vi "NI OCR-Detect Characters Setting.vi"(8 "error in":errorcluster, 11 "Buffer Data In":T3={"VI Refnum"=refnum, "Src Image"="NI OCR-Src Image", "Dst Image"="NI OCR-Dst Image", "Ctl Refnum []"=[refnum, refnum, refnum], "Ctl Label"=["Detect Characters", "Display Image", "Import Picture"], "User Event"=refnum, "Event Registration Refnum"=refnum, "Timeout"=-1, "IMAQ OCR Session"=refnum, "Objects"=[], "ROI Descriptor"={"Global Rectangle"=[], "Contours"=[]}, "Settings"={"Objects"=0, "Threshold"=128, "Reject Border"=FALSE, "Fill Holes"=FALSE, "Min Object Size"=FALSE, "Min Size"=3, "Max Object Size"=FALSE, "Max Size"=100, "Show Search Area"=FALSE, "Show Center"=TRUE, "Show Bounding Box"=TRUE}} {"Settings"."Objects" items=["Bright Objects", "Dark Objects"]; "Settings"."Threshold" min=1 max=999999999 step=1; "Settings"."Max Size" min=1 max=999999999 step=1; "Settings"."Min Size" min=1 max=999999999 step=1; "ROI Descriptor"."Contours"."Type" items=["No Selection", "Point", "Line", "Rectangle", "Oval", "Polygon", "Freehand Region", "Annulus", "Unused2", "Unused3", "Broken Line", "Freehand Line", "Rotated Rectangle"]; "Objects"."Aspect Ratio" format="%.2f"; "Objects"."Orientation" format="%.2f"; "Objects"."Area" format="%.2f"; "Objects"."Object Center"."Y" format="%.2f"; "Objects"."Object Center"."X" format="%.2f"}) -> (0 "error out":errorcluster, 2 "OK?":bool, 3 "Buffer Data Out":T3={"VI Refnum"=refnum, "Src Image"="NI OCR-Src Image", "Dst Image"="NI OCR-Dst Image", "Ctl Refnum []"=[refnum, refnum, refnum], "Ctl Label"=["Detect Characters", "Display Image", "Import Picture"], "User Event"=refnum, "Event Registration Refnum"=refnum, "Timeout"=-1, "IMAQ OCR Session"=refnum, "Objects"=[{"Object Center"={"X"=111.53468, "Y"=84.57803}, "Bounding Box"={"X Left"=95, "Y Top"=62, "X Right"=124, "Y Bottom"=108}, "Area"=692.0, "Orientation"=88.71199, "Aspect Ratio"=0.6304348, "Nb Holes"=0}, {"Object Center"={"X"=74.43038, "Y"=89.12658}, "Bounding Box"={"X Left"=60, "Y Top"=64, "X Right"=89, "Y Bottom"=110}, "Area"=632.0, "Orientation"=97.4022, "Aspect Ratio"=0.6304348, "Nb Holes"=0}, {"Object Center"={"X"=147.98517, "Y"=88.570015}, "Bounding Box"={"X Left"=132, "Y Top"=66, "X Right"=160, "Y Bottom"=112}, "Area"=607.0, "Orientation"=87.522575, "Aspect Ratio"=0.6086956, "Nb Holes"=0}, {"Object Center"={"X"=179.27258, "Y"=95.40412}, "Bounding Box"={"X Left"=168, "Y Top"=68, "X Right"=197, "Y Bottom"=114}, "Area"=631.0, "Orientation"=112.89326, "Aspect Ratio"=0.6304348, "Nb Holes"=1}, {"Object Center"={"X"=271.875, "Y"=72.375}, "Bounding Box"={"X Left"=270, "Y Top"=69, "X Right"=274, "Y Bottom"=78}, "Area"=24.0, "Orientation"=99.49205, "Aspect Ratio"=0.44444445, "Nb Holes"=0}, {"Object Center"={"X"=217.32158, "Y"=92.65162}, "Bounding Box"={"X Left"=203, "Y Top"=70, "X Right"=232, "Y Bottom"=116}, "Area"=709.0, "Orientation"=79.66425, "Aspect Ratio"=0.6304348, "Nb Holes"=0}, {"Object Center"={"X"=248.96008, "Y"=100.51471}, "Bounding Box"={"X Left"=241, "Y Top"=73, "X Right"=269, "Y Bottom"=118}, "Area"=476.0, "Orientation"=108.11947, "Aspect Ratio"=0.62222224, "Nb Holes"=0}], "ROI Descriptor"={"Global Rectangle"=[], "Contours"=[]}, "Settings"={"Objects"=0, "Threshold"=128, "Reject Border"=FALSE, "Fill Holes"=FALSE, "Min Object Size"=FALSE, "Min Size"=3, "Max Object Size"=FALSE, "Max Size"=100, "Show Search Area"=FALSE, "Show Center"=TRUE, "Show Bounding Box"=TRUE}} {"Settings"."Objects" items=["Bright Objects", "Dark Objects"]; "Settings"."Threshold" min=1 max=999999999 step=1; "Settings"."Max Size" min=1 max=999999999 step=1; "Settings"."Min Size" min=1 max=999999999 step=1; "ROI Descriptor"."Contours"."Type" items=["No Selection", "Point", "Line", "Rectangle", "Oval", "Polygon", "Freehand Region", "Annulus", "Unused2", "Unused3", "Broken Line", "Freehand Line", "Rotated Rectangle"]; "Objects"."Aspect Ratio" format="%.2f"; "Objects"."Orientation" format="%.2f"; "Objects"."Area" format="%.2f"; "Objects"."Object Center"."Y" format="%.2f"; "Objects"."Object Center"."X" format="%.2f"})   [LabVIEW 2016]
uses:
  Data Def/NI OCR-Buffer Data.ctl
  <vilib>/vision/Image Controls.llb/IMAQ Image.ctl
  Data Def/NI OCR-User Event Data.ctl
  <vilib>/vision/OCR.llb/IMAQ OCR Session.ctl
  <vilib>/Utility/miscctls.llb/LVPointTypeDef.ctl
  Data Def/NI OCR-Detect Characters State.ctl
panel:
  in  "Cancel":bool
  in  "OK":bool
  in  "Setting":T1={"Objects"=1, "Threshold"=128.0, "Ignore Objects touching Image Borders"=FALSE, "Fill Holes within Objects"=FALSE, "Minimum Object Size"=FALSE, "Min Size(Pixels)"=0.0, "Maximum Object Size"=FALSE, "Max Size(Pixels)"=1000.0, "Show Search Area"=TRUE, "Show Center"=TRUE, "Show Bounding Box"=TRUE} {"Objects" items=["Bright Objects", "Dark Objects"]}
  out "Display Image":T2(plugin-control)
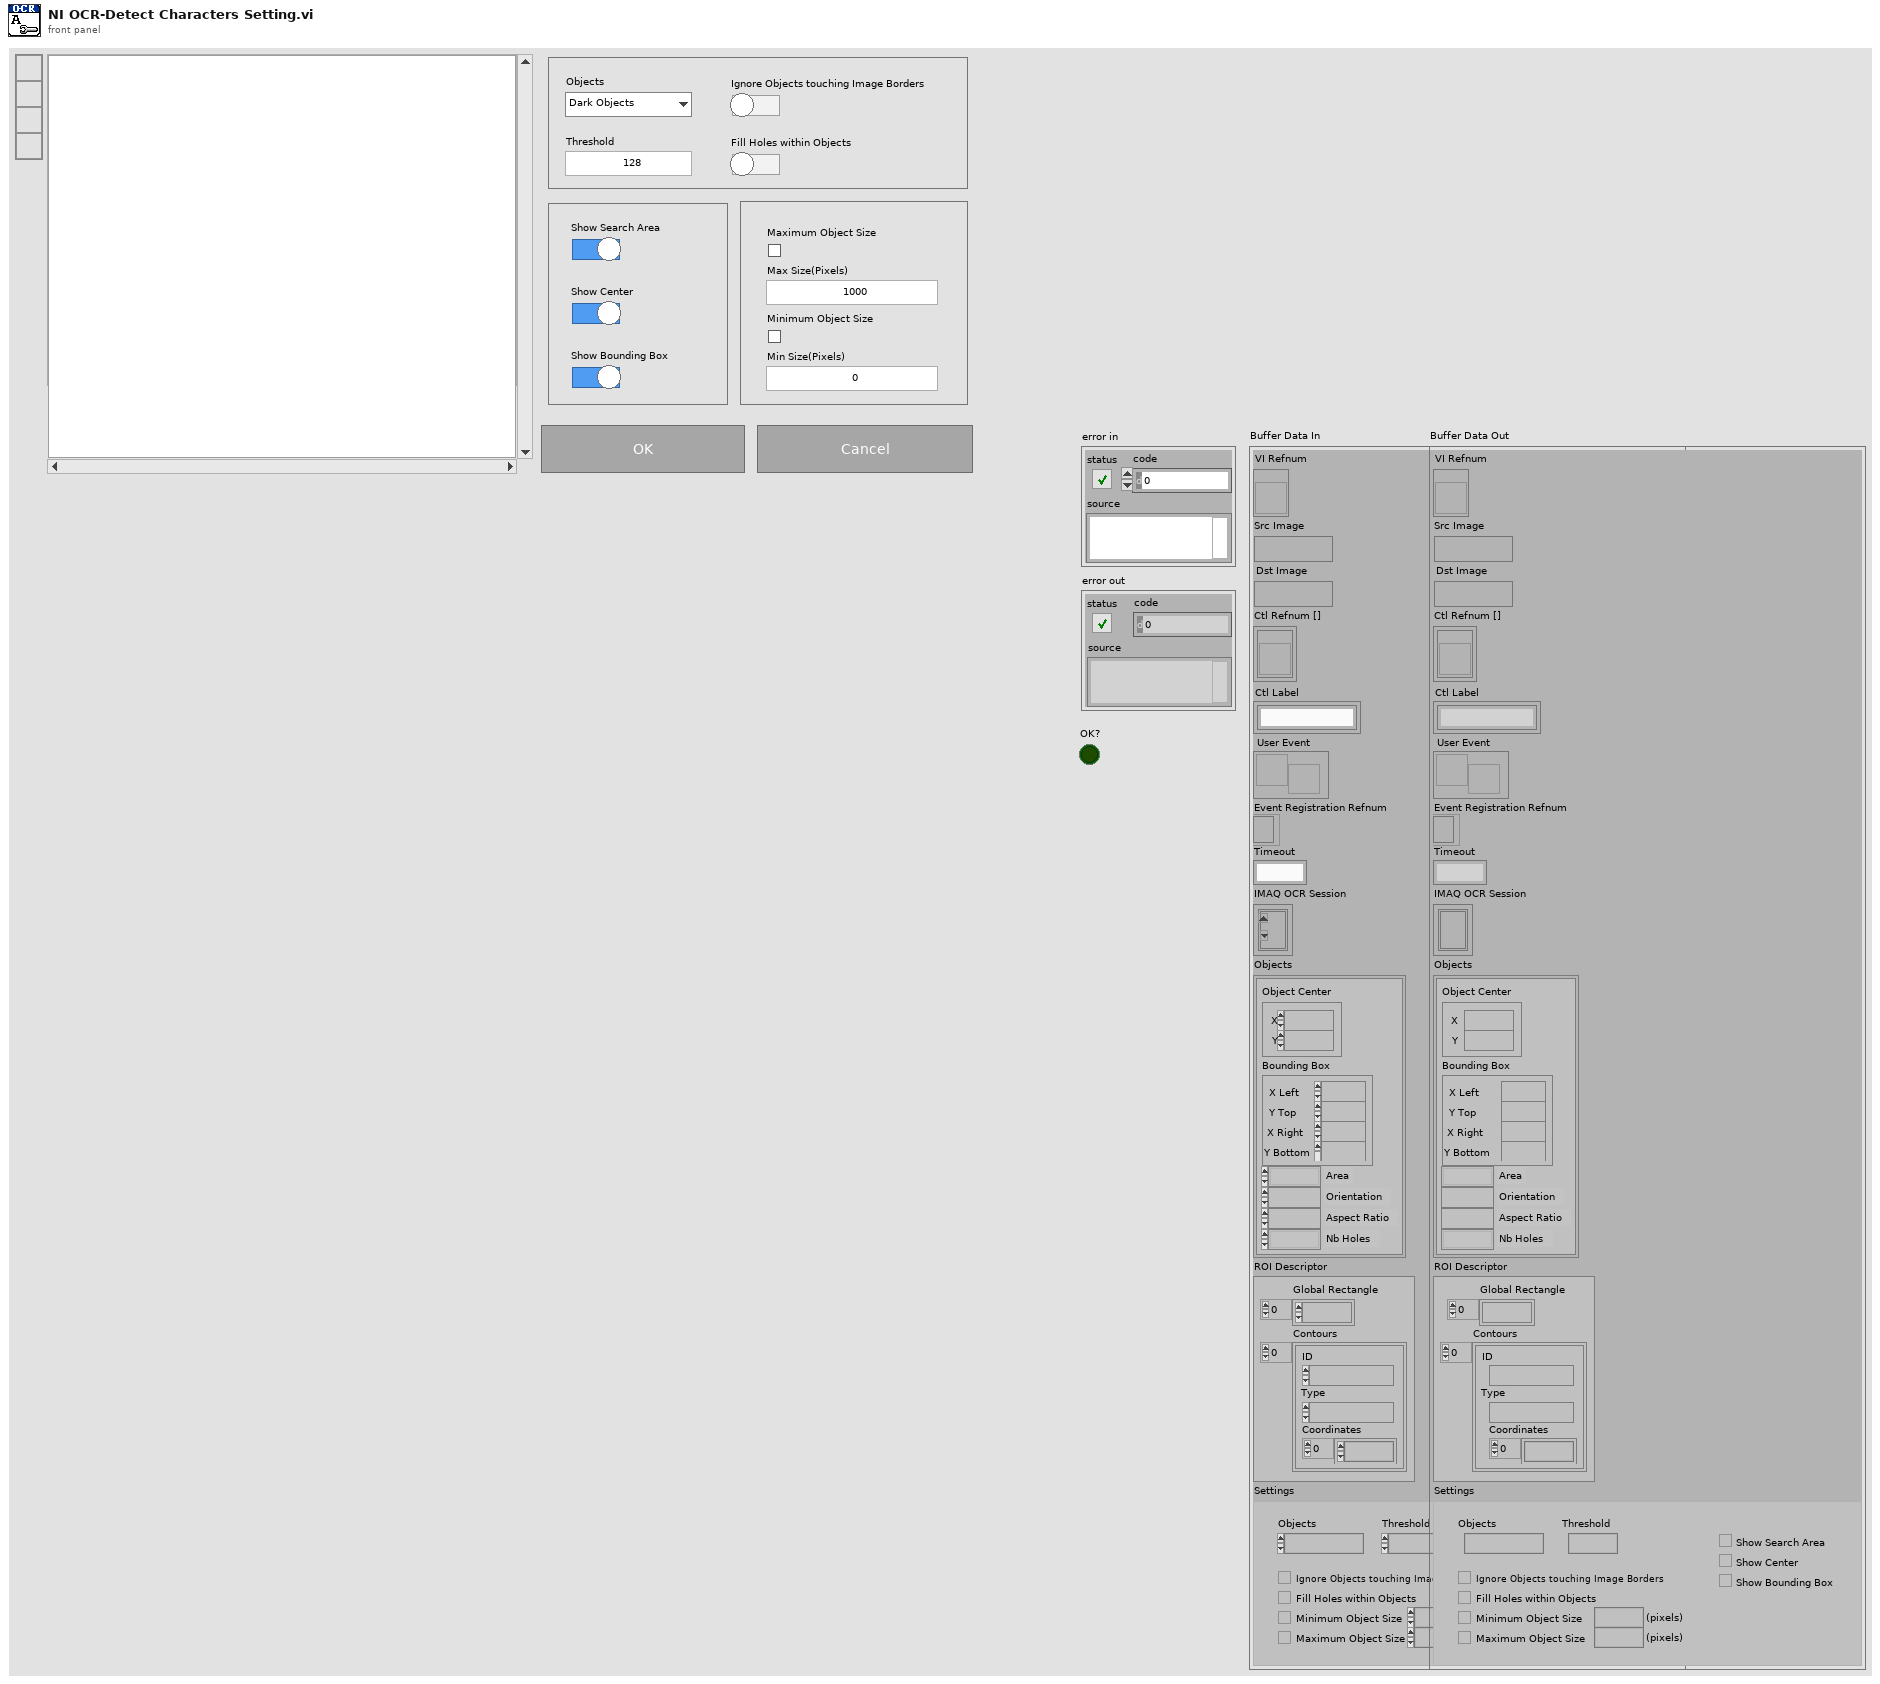
[diagram p1: front panel]
types:
  T1 = cluster{"Objects":u16, "Threshold":dbl, "Ignore Objects touching Image Borders":bool, "Fill Holes within Objects":bool, "Minimum Object Size":bool, "Min Size(Pixels)":dbl, "Maximum Object Size":bool, "Max Size(Pixels)":dbl, "Show Search Area":bool, "Show Center":bool, "Show Bounding Box":bool}
  T2 = typedef "IMAQ Image.ctl" = refnum<image>
  T3 = typedef "NI OCR-Buffer Data.ctl" = cluster{"VI Refnum":refnum<vi>, "Src Image":T2, "Dst Image":T2, "Ctl Refnum []":refnum<vi>[], "Ctl Label":string[], "User Event":refnum<user-event>, "Event Registration Refnum":refnum<event-registration>, "Timeout":i32, "IMAQ OCR Session":T4, "Objects":cluster{"Object Center":cluster{"X":sgl, "Y":sgl}, "Bounding Box":cluster{"X Left":i32, "Y Top":i32, "X Right":i32, "Y Bottom":i32}, "Area":sgl, "Orientation":sgl, "Aspect Ratio":sgl, "Nb Holes":i32}[], "ROI Descriptor":T5, "Settings":cluster{"Objects":u16, "Threshold":i32, "Reject Border":bool, "Fill Holes":bool, "Min Object Size":bool, "Min Size":i32, "Max Object Size":bool, "Max Size":i32, "Show Search Area":bool, "Show Center":bool, "Show Bounding Box":bool}}
  T4 = typedef "IMAQ OCR Session.ctl" = refnum<k1>
  T5 = typedef "ROI Descriptor" = cluster{"Global Rectangle":i32[], "Contours":cluster{"ID":enum32{"External", "Internal"}, "Type":u32, "Coordinates":i32[]}[]}
  T6 = typedef "NI OCR-Detect Characters State.ctl" = enum16{"Detect", "Event", "Stop"}
  T7 = typedef "LVPointTypeDef.ctl" = cluster{"Horizontal":i16, "Vertical":i16}
  T8 = cluster{"Global Rectangle":i32[], "Contours":cluster{"Contour Type":u32, "ROI Type":u32, "Points":i32[]}[]}
  T9 = typedef "IMAQ Rectangle" = cluster{"Left":i32, "Top":i32, "Right":i32, "Bottom":i32, "Rotation":dbl}
  T10 = cluster{"Object Center":cluster{"X":sgl, "Y":sgl}, "Bounding Box":cluster{"X Left":i32, "Y Top":i32, "X Right":i32, "Y Bottom":i32}, "Area":sgl, "Orientation":sgl, "Aspect Ratio":sgl, "Nb Holes":i32}[]
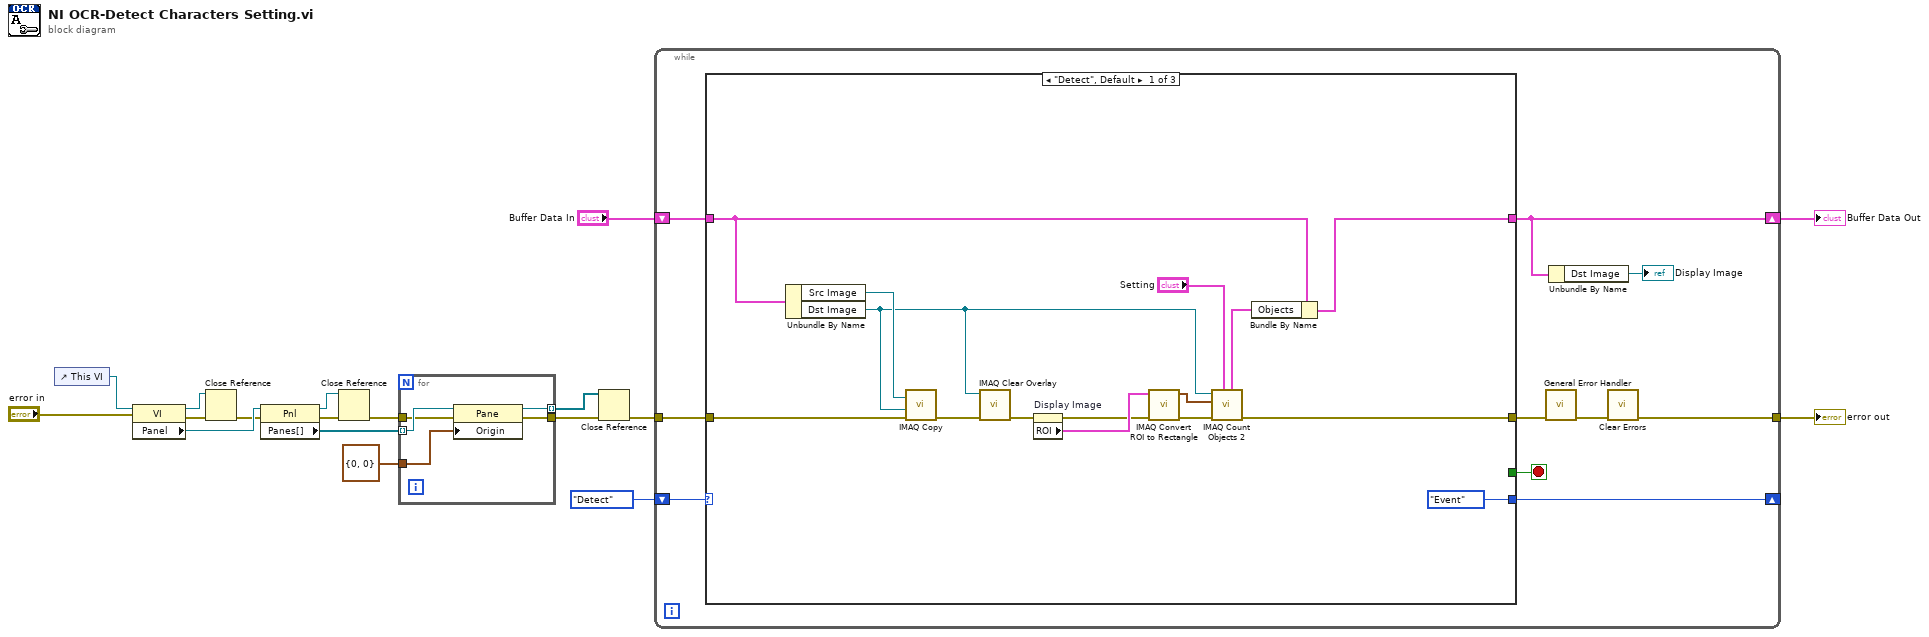
[diagram p0: block diagram]
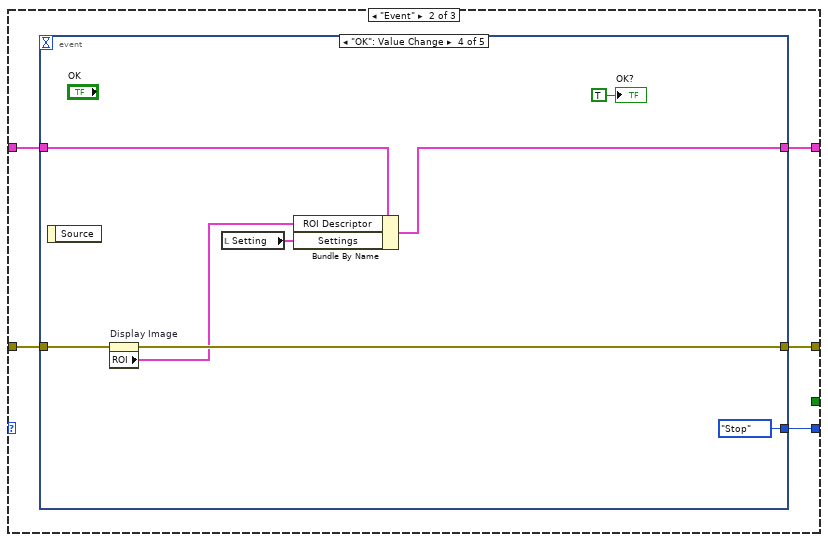
[diagram p2: hidden frame]
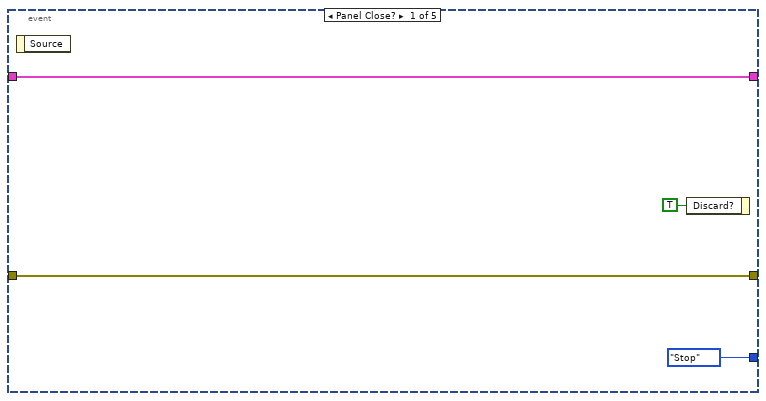
[diagram p3: hidden frame]
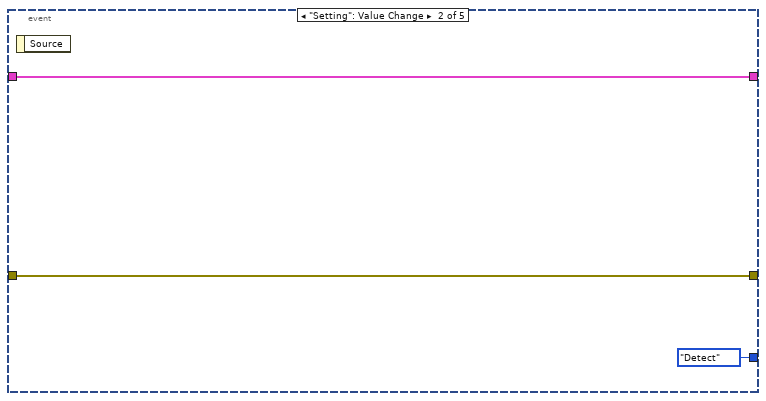
[diagram p4: hidden frame]
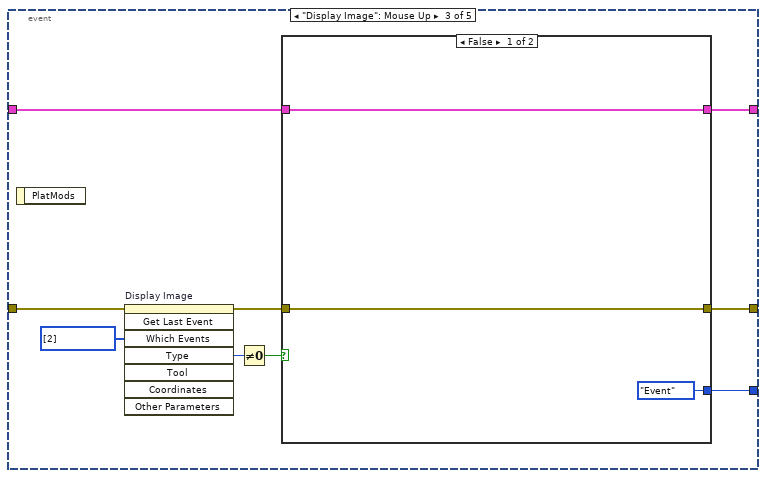
[diagram p5: hidden frame]
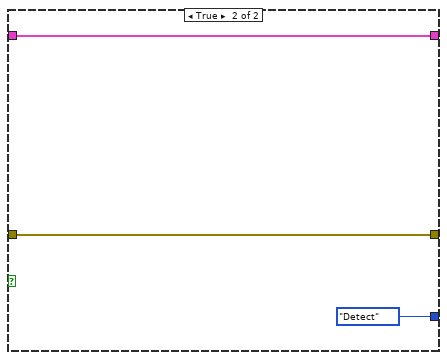
[diagram p6: hidden frame]
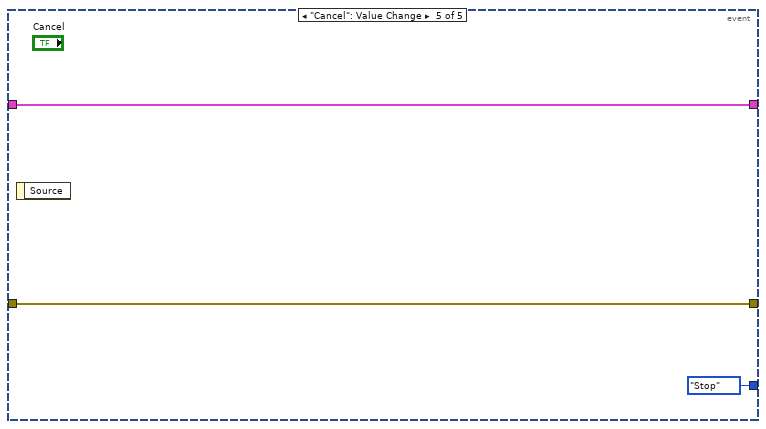
[diagram p7: hidden frame]
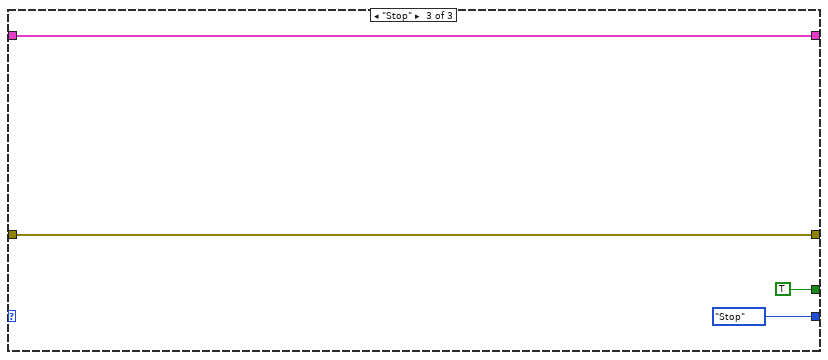
[diagram p8: hidden frame]
diagram:
  n1 = control-ref of="This VI"() -> (w12:refnum<vi>)
  n2 = property class="VI"(reference=w12, error in="error in") -> (reference out=w10:refnum<vi>, error out=w11:errorcluster, "Panel"=w18:refnum<vi>)
  n3 = Close Reference(reference=w10, error in (no error)=w11) -> (error out=w9:errorcluster)
  n4 = property class="Pnl"(reference=w18, error in=w9) -> (reference out=w14:refnum<vi>, error out=w15:errorcluster, "Panes[]"=w17:refnum<vi>[])
  n5 = Close Reference(reference=w14, error in (no error)=w15) -> (error out=w13:errorcluster)
  n6 = for {
    tunnel: w13 -> [w22]
    tunnel: w17 -> [w23] mode=indexing
    tunnel: T7 {"Horizontal"=0, "Vertical"=0} ("Origin") -> [w21]
    tunnel: [w20] -> w8
    tunnel: [w19] -> w7 mode=indexing
    n7 = property class="Pane"(reference=w23, error in=w22, "Origin"=w21) -> (reference out=w19:refnum<vi>, error out=w20:errorcluster)
  }
  n8 = Close Reference(reference=w7, error in (no error)=w8) -> (error out=w5:errorcluster)
  n9 = while {
    shift-right: [w28] -> _
    shift-left: NI_OCR-Detect_Characters_State."Detect" ("Detect Characters State") -> [w33]
    tunnel: w5 -> [w32]
    shift-right: [w30] -> w1
    shift-left: "Buffer Data In" -> [w31]
    tunnel: [w24] -> w2
    stop <- w27 stop-if-true
    n10 = case shown="\"Detect\", Default" w33 {
      tunnel: w32 -> [w48 w51 w90]
      tunnel: w31 -> [w36 w53 w87]
      tunnel: [w34 w52 w87] -> w30
      tunnel: [w39 w50 w90] -> w26
      tunnel: [NI_OCR-Detect_Characters_State."Event" ("Detect Characters State") w49 NI_OCR-Detect_Characters_State."Stop" ("Detect Characters State")] -> w28
      tunnel: [_ _ TRUE] -> w27
      frame "Detect", Default {
        n11 = Unbundle By Name(w36) -> ("Src Image"=w47:T2, "Dst Image"=w37:T2)
        n12 = call "IMAQ Copy"("error in (no error)"=w48, "Image Dst"=w37, "Image Src"=w47) -> ("error out"=w40:errorcluster)  [unwired: 3 in, 1 out]
        n13 = call "IMAQ Clear Overlay"("error in (no error)"=w40, "Image"=w37) -> ("error out"=w45:errorcluster)  [unwired: 8 in, 1 out]
        n14 = property on="Display Image" class="ImageControl"(error in=w45) -> (error out=w41:errorcluster, "ROI"=w42:T8)  [unwired: 1 in, 1 out]
        n15 = call "IMAQ Convert ROI to Rectangle"("error in (no error)"=w41, "ROI Descriptor"=w42) -> ("error out"=w43:errorcluster, "Rectangle"=w44:T9)  [unwired: 7 in]
        n16 = call "IMAQ Count Objects 2"("Settings"="Setting", "error in (no error)"=w43, "Search Rect (entire image)"=w44, "Image"=w37) -> ("error out"=w39:errorcluster, "Objects"=w35:T10)  [unwired: 3 in, 3 out]
        n17 = Bundle By Name(cluster=w36, "Objects"=w35) -> (w34:T3)
      }
      frame "Event" {
        n18 = event shown="[3] \"OK\": Value Change" {
          selector: _ -> [_ _ _ _ _]
          dyn-events: _ -> [_ _ _ _ _]
          timeout: _ -> [_ _ _ _ _]
          tunnel: w53 -> [w57 w60 w66 w81 w86]
          tunnel: [w57 w60 w63 w76 w86] -> w52
          tunnel: w51 -> [w56 w59 w69 w80 w85]
          tunnel: [w56 w59 w61 w79 w85] -> w50
          tunnel: [NI_OCR-Detect_Characters_State."Stop" ("Detect Characters State") NI_OCR-Detect_Characters_State."Detect" ("Detect Characters State") w62 NI_OCR-Detect_Characters_State."Stop" ("Detect Characters State") NI_OCR-Detect_Characters_State."Stop" ("Detect Characters State")] -> w49
          event Panel Close? {
            n19 = event-data() -> ()  [unwired: 1 in, 1 out]
            n20 = event-data("Discard?"=TRUE) -> ()  [unwired: 1 in, 1 out]
          }
          event "Setting": Value Change {
            n21 = event-data() -> ()  [unwired: 1 in, 1 out]
          }
          event "Display Image": Mouse Up {
            w68 = i32[] [2] items=["No Event"=0, "Click Event"=1, "Draw Event"=2, "Size Event"=4, "Scroll Event"=5, "Double Click Event"=8] ("Which Events")
            n22 = event-data() -> ()  [unwired: 1 in, 1 out]
            n23 = invoke on="Display Image" class="ImageControl" method="Get Last Event"(error in=w69, "Which Events"=w68) -> (error out=w67:errorcluster, "Type"=w65:i32)  [unwired: 6 in, 6 out]
            n24 = Not Equal To 0?(x=w65) -> (x != 0?=w64:bool)
            n25 = case shown="False" w64 {
              tunnel: w67 -> [w71 w73]
              tunnel: w66 -> [w72 w75]
              tunnel: [w72 w75] -> w63
              tunnel: [NI_OCR-Detect_Characters_State."Event" ("Detect Characters State") NI_OCR-Detect_Characters_State."Detect" ("Detect Characters State")] -> w62
              tunnel: [w71 w73] -> w61
              frame False {
              }
              frame True {
              }
            }
          }
          event "OK": Value Change {
            n26 = event-data() -> ()  [unwired: 1 in, 1 out]
            n27 = property on="Display Image" class="ImageControl"(error in=w80) -> (error out=w79:errorcluster, "ROI"=w78:T8)  [unwired: 1 in, 1 out]
            n28 = local read "Setting"() -> (w77:T1)
            n29 = Bundle By Name(cluster=w81, "ROI Descriptor"=w78, "Settings"=w77) -> (w76:T3)
            "OK?" <- TRUE ("OK?")
          }
          event "Cancel": Value Change {
            n30 = event-data() -> ()  [unwired: 1 in, 1 out]
          }
        }
      }
      frame "Stop" {
      }
    }
    n31 = call <vilib>:"General Error Handler.vi"("error in (no error)"=w26) -> ("error out"=w25:errorcluster)  [unwired: 10 in, 4 out]
    n32 = Unbundle By Name(w30) -> ("Dst Image"=→"Display Image":T2)
    n33 = call <vilib>:"Clear Errors.vi"("error in (no error)"=w25) -> ("error out"=w24:errorcluster)  [unwired: 5 in, 1 out]
  }
  "error out" <- w2
  "Buffer Data Out" <- w1
